vi "Allocate Image Memory (Pattern).vi"() -> (0 "error out":errorcluster, 1 "Template Patterns":T1[](array[typedef]), 2 "Process Memory":T1, 3 "Acquisition Memory":T1[](array[typedef]))   [LabVIEW 2018]
uses:
  <vilib>/vision/Image Controls.llb/IMAQ Image.ctl
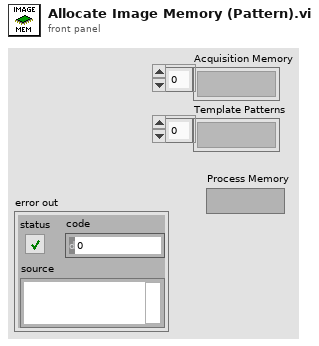
[diagram p1: front panel]
types:
  T1 = typedef "IMAQ Image.ctl" = refnum<image>
  T2 = typedef "Image Type" = u32
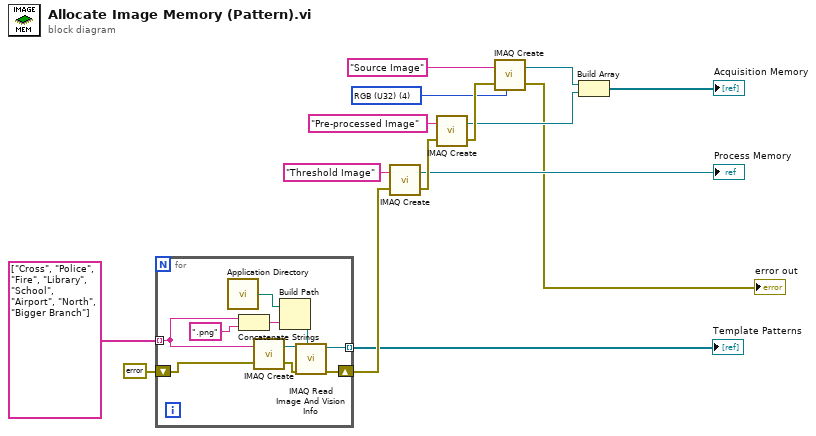
[diagram p0: block diagram]
diagram:
  w6 = T2 4 items=["Grayscale (U8)", "Grayscale (I16)", "Grayscale (SGL)", "Complex (CSG)", "RGB (U32)", "HSL (U32)", "RGB (U64)", "Grayscale (U16)"] ("Image Type")
  n1 = for {
    tunnel: string[] ["Cross", "Police", "Fire", "Library", "School", "Airport", "North", "Bigger Branch"] -> [w21] mode=indexing
    shift-right: [w18] -> w3
    shift-left: errorcluster {"status"=FALSE, "code"=0, "source"=""} ("error out") -> [w17]
    tunnel: [w16] -> w2 mode=indexing
    n2 = call <vilib>:"Application Directory.vi"() -> ("Application Directory"=w23:path)
    n3 = Concatenate Strings(w21, ".png" ("string")) -> (w22:string)
    n4 = call "IMAQ Create"("Image Name"=w21, "error in (no error)"=w17) -> ("New Image"=w25:T1, "error out"=w19:errorcluster)  [unwired: 3 in]
    n5 = Build Path(base path=w23, name or relative path=w22) -> (appended path=w24:path)
    n6 = call "IMAQ Read Image And Vision Info"("File Path"=w24, "error in (no error)"=w19, "Image"=w25) -> ("error out"=w18:errorcluster, "Image Out"=w16:T1)  [unwired: 6 in, 1 out]
  }
  "Template Patterns" <- w2
  n7 = call "IMAQ Create"("Image Name"="Threshold Image", "error in (no error)"=w3) -> ("New Image"=→"Process Memory":T1, "error out"=w13:errorcluster)  [unwired: 3 in]
  n8 = call "IMAQ Create"("Image Name"="Pre-processed Image", "error in (no error)"=w13) -> ("New Image"=w9:T1, "error out"=w10:errorcluster)  [unwired: 3 in]
  n9 = call "IMAQ Create"("Image Name"="Source Image", "Image Type"=w6, "error in (no error)"=w10) -> ("New Image"=w8:T1, "error out"=→"error out":errorcluster)  [unwired: 2 in]
  n10 = Build Array(w8, w9) -> (→"Acquisition Memory":T1[])
